vi "generate_DAC_voltages_flexRIO.vi"(7 "focus mode?":bool, 8 "derived values":T1, 9 "scan specification":T4={"x amplitude"=0, "x resolution (pixels)"=0, "x offset fly-forward (iterations)"=0, "x offset fly-back (iterations)"=0, "y resolution (nr. of lines)"=0, "y step size"=0, "iterations per pixel"=0, "number of frames"=0, "y offset (pixels)"=0, "number of y-brake lines  (before y-fly-back)"=0, "number y-brake lines (after y-fly-back)"=0, "number of y-fly-back steps"=8, "lines per z step"=0, "number of z/intensity tuples"=0, "number of repetitions (volumes or planes)"=0}, 10 "counter cluster in":T2, 11 "resonant trigger":bool) -> (0 "acquire?":bool, 1 "fly-back acquisition phase?":bool, 2 "counter cluster out":T2, 3 "DAC voltages":T3 {"ch6" max=4095 step=1; "ch5" max=4095 step=1; "ch4" max=4095 step=1; "ch3" max=4095 step=1; "ch2" max=4095 step=1; "ch1" max=4095 step=1; "ch0" max=4095 step=1})   [LabVIEW 2010]
uses:
  scan_specification_cluster_flexRIO.ctl
  DAC_voltage_cluster_flexRIO.ctl
  counter_cluster_flexRIO.ctl
  derived_values_cluster_flexRIO.ctl
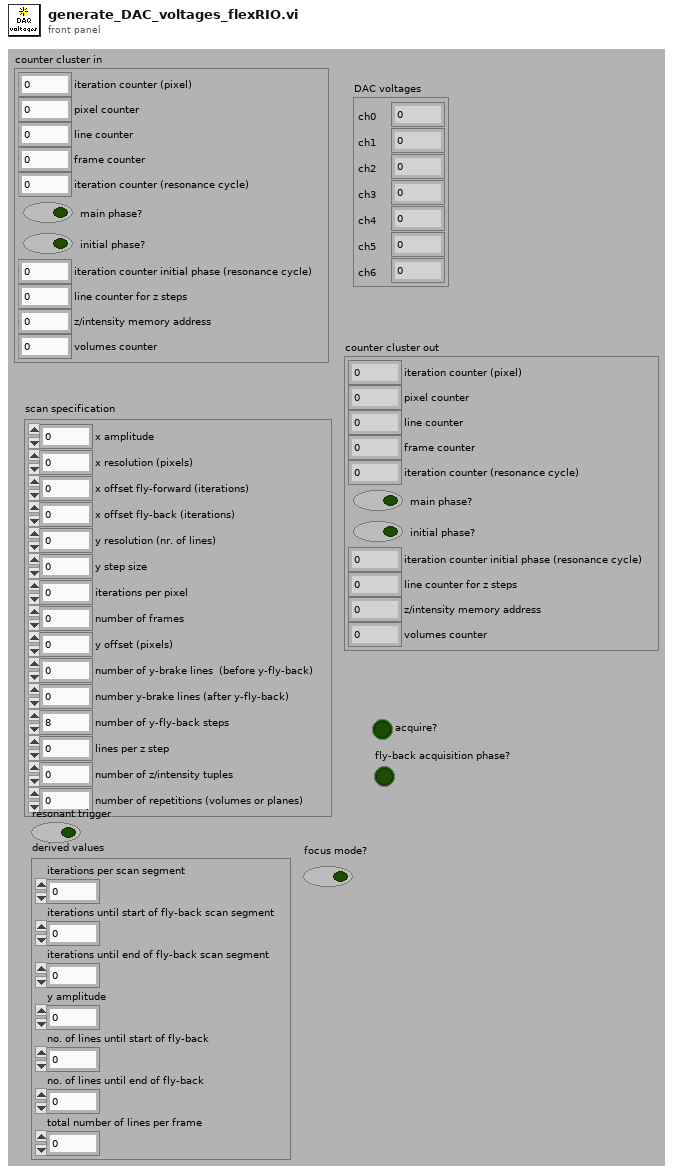
[diagram p1: front panel]
types:
  T1 = typedef "derived_values_cluster_flexRIO.ctl" = cluster{"iterations per scan segment":u16, "iterations until start of fly-back scan segment":u16, "iterations until end of fly-back scan segment":u16, "y amplitude":u16, "no. of lines until start of fly-back":u16, "no. of lines until end of fly-back":u16, "total number of lines per frame ":u16}
  T2 = typedef "counter_cluster_flexRIO.ctl" = cluster{"iteration counter (pixel)":u16, "pixel counter":u16, "line counter":u16, "frame counter":u16, "iteration counter (resonance cycle)":u16, "main phase?":bool, "initial phase?":bool, "iteration counter initial phase (resonance cycle)":u16, "line counter for z steps":u16, "z/intensity memory address":u32, "volumes counter":u16}
  T3 = typedef "DAC_voltage_cluster_flexRIO.ctl" = cluster{"ch0":u16, "ch1":u16, "ch2":u16, "ch3":u16, "ch4":u16, "ch5":u16, "ch6":u16}
  T4 = typedef "scan_specification_cluster_flexRIO.ctl" = cluster{"x amplitude":u16, "x resolution (pixels)":u16, "x offset fly-forward (iterations)":u16, "x offset fly-back (iterations)":u16, "y resolution (nr. of lines)":u16, "y step size":u16, "iterations per pixel":u16, "number of frames":i32, "y offset (pixels)":u16, "number of y-brake lines  (before y-fly-back)":u16, "number y-brake lines (after y-fly-back)":u16, "number of y-fly-back steps":u16, "lines per z step":u16, "number of z/intensity tuples":u16, "number of repetitions (volumes or planes)":i32}
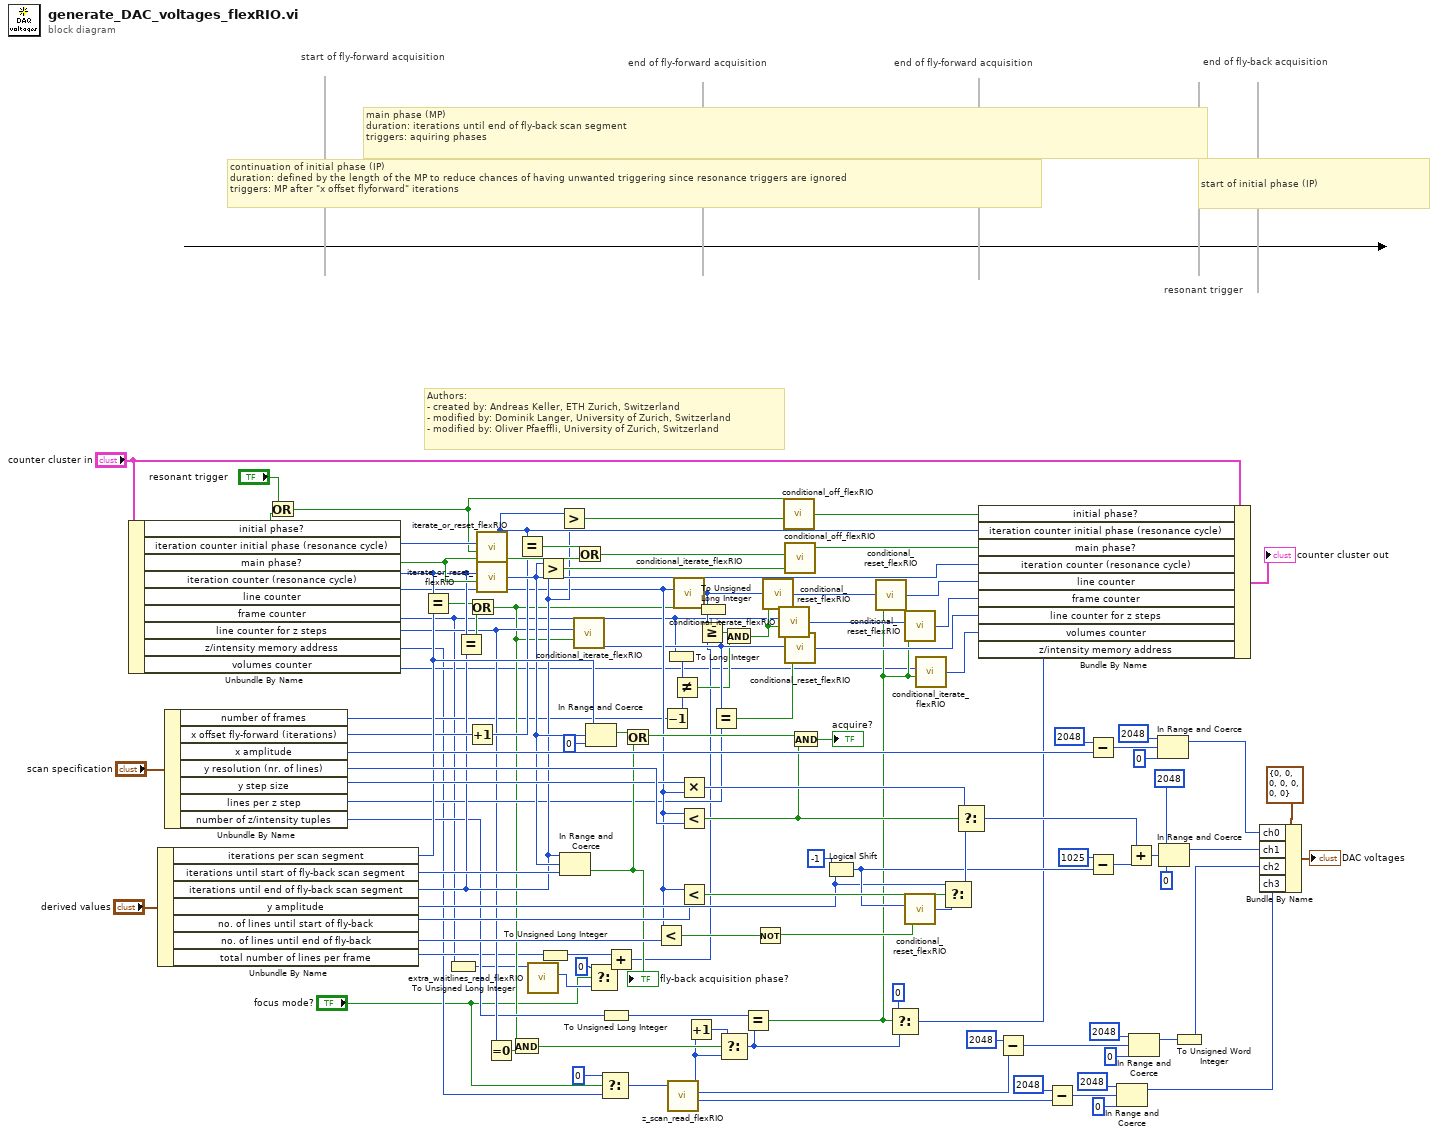
[diagram p0: block diagram]
diagram:
  # "start of initial phase (IP)"
  # "continuation of initial phase (IP)\nduration: defined by the length of the MP to reduce chances of having unwanted triggering since resonance triggers are ignored\ntriggers: MP after \"x offset flyforward\" iterations"
  # "end of fly-back acquisition"
  # "end of fly-forward acquisition"
  # "end of fly-forward acquisition"
  # "start of fly-forward acquisition"
  # "main phase (MP)\nduration: iterations until end of fly-back scan segment\ntriggers: aquiring phases"
  # "resonant trigger"
  # "Authors: \n- created by: Andreas Keller, ETH Zurich, Switzerland\n- modified by: Dominik Langer, University of Zurich, Switzerland\n- modified by: Oliver Pfaeffli, University of Zurich, Switzerland"
  n1 = Unbundle By Name("counter cluster in") -> ("initial phase?"=w85:bool, "iteration counter initial phase (resonance cycle)"=w81:u16, "main phase?"=w80:bool, "iteration counter (resonance cycle)"=w63:u16, "line counter"=w60:u16, "frame counter"=w14:u16, "line counter for z steps"=w53:u16, "z/intensity memory address"=w5:u32, "volumes counter"=w7:u16)
  n2 = Unbundle By Name("derived values") -> ("iterations per scan segment"=w83:u16, "iterations until start of fly-back scan segment"=w87:u16, "iterations until end of fly-back scan segment"=w62:u16, "y amplitude"=w69:u16, "no. of lines until start of fly-back"=w68:u16, "no. of lines until end of fly-back"=w86:u16, "total number of lines per frame"=w29:u16)
  n3 = Unbundle By Name("scan specification") -> ("number of frames"=w17:i32, "x offset fly-forward (iterations)"=w67:u16, "x amplitude"=w96:u16, "y resolution (nr. of lines)"=w93:u16, "y step size"=w92:u16, "lines per z step"=w57:u16, "number of z/intensity tuples"=w51:u16)
  n4 = Or(x="resonant trigger", y=w85) -> (x .or. y?=w77:bool)
  n5 = Equal?(x=w63, y=w83) -> (x = y?=w58:bool)
  n6 = To Unsigned Long Integer(number=w14) -> (unsigned 32bit integer=w30:u32)
  n7 = Equal?(x=w63, y=w62) -> (x = y?=w61:bool)
  n8 = Increment(x=w67) -> (x+1=w66:u16)
  n9 = Or(x=w58, y=w61) -> (x .or. y?=w35:bool)
  n10 = call "iterate_or_reset_flexRIO.vi"("iterate?"=w77, "number in"=w81) -> ("number out"=w64:u16)  [unwired: 4 in]
  n11 = call "iterate_or_reset_flexRIO.vi"("iterate?"=w80, "number in"=w63) -> ("number out"=w79:u16)  [unwired: 4 in]
  n12 = Equal To 0?(x=w53) -> (x = 0?=w36:bool)
  n13 = And(x=w35, y=w36) -> (x .and. y?=w34:bool)
  n14 = Equal?(x=w64, y=w66) -> (x = y?=w78:bool)
  n15 = call "extra_waitlines_read_flexRIO.vi"("address extra waitlines IN"=w30) -> ("extra waitline data"=w10:u32)  [unwired: 9 in, 1 out]
  n16 = Greater?(x=w79, y=w62) -> (0:w75:bool)
  n17 = To Unsigned Long Integer(number=w29) -> (unsigned 32bit integer=w28:u32)
  n18 = Greater?(x=w64, y=w62) -> (0:w65:bool)
  n19 = In Range and Coerce(upper limit=w62, x=w79, lower limit=w87) -> (In Range?=w59:bool)  [unwired: 1 out]
  "fly-back acquisition phase?" <- w59
  n20 = call "conditional_iterate_flexRIO.vi"("iterate?"=w35, "number in"=w53) -> ("number out"=w54:u16)  [unwired: 4 in]
  n21 = Or(x=w78, y=w80) -> (x .or. y?=w74:bool)
  n22 = In Range and Coerce(upper limit=w83, x=w79, lower limit=u16 0) -> (In Range?=w108:bool)  [unwired: 1 out]
  n23 = Select(t=u32 0, s="focus mode?", f=w10) -> (s? t:f=w9:u32)
  n24 = Select(t=u32 0, s="focus mode?", f=w5) -> (s? t:f=w4:u32)
  n25 = To Unsigned Long Integer(number=w51) -> (unsigned 32bit integer=w50:u32)
  n26 = Add(x=w28, y=w9) -> (x+y=w11:u32)
  n27 = Or(x=w108, y=w59) -> (x .or. y?=w91:bool)
  n28 = Less?(x=w60, y=w86) -> (x < y?=w89:bool)
  n29 = Decrement(x=w17) -> (x-1=w16:i32)
  n30 = To Long Integer(number=w14) -> (32bit integer=w13:i32)
  n31 = call "z_scan_read_flexRIO.vi"("address in"=w4) -> ("intensity"=w33:u16, "z-value"=w31:i16, "address out"=w32:u32)  [unwired: 8 in]
  n32 = Not Equal?(x=w13, y=w16) -> (x != y?=w15:bool)
  n33 = call "conditional_iterate_flexRIO.vi"("iterate?"=w35, "number in"=w60) -> ("number out"=w27:u16)  [unwired: 4 in]
  n34 = Multiply(x=w92, y=w60) -> (x*y=w112:u16)
  n35 = Less?(x=w60, y=w93) -> (x < y?=w90:bool)
  n36 = Less?(x=w60, y=w68) -> (x < y?=w114:bool)
  n37 = Increment(x=w32) -> (x+1=w52:u32)
  n38 = To Unsigned Long Integer(number=w27) -> (unsigned 32bit integer=w26:u32)
  n39 = Greater Or Equal?(x=w26, y=w11) -> (x >= y?=w19:bool)
  n40 = Equal?(x=w54, y=w57) -> (x = y?=w55:bool)
  n41 = Select(t=w52, s=w34, f=w32) -> (s? t:f=w49:u32)
  n42 = And(x=w19, y=w15) -> (x .and. y?=w18:bool)
  n43 = Equal?(x=w50, y=w49) -> (x = y?=w12:bool)
  n44 = Not(x=w89) -> (.not. x?=w71:bool)
  n45 = call "conditional_reset_flexRIO.vi"("reset?"=w18, "number in"=w27) -> ("number out"=w21:u16)  [unwired: 4 in]
  n46 = call "conditional_iterate_flexRIO.vi"("iterate?"=w18, "number in"=w14) -> ("number out"=w23:u16)  [unwired: 4 in]
  n47 = call "conditional_off_flexRIO.vi"("switch off?"=w65, "boolean in"=w77) -> ("boolean out"=w76:bool)  [unwired: 4 in]
  n48 = call "conditional_off_flexRIO.vi"("switch off?"=w75, "boolean in"=w74) -> ("boolean out"=w73:bool)  [unwired: 4 in]
  n49 = call "conditional_reset_flexRIO.vi"("reset?"=w55, "number in"=w54) -> ("number out"=w56:u16)  [unwired: 4 in]
  n50 = And(x=w91, y=w90) -> (x .and. y?=→"acquire?":bool)
  n51 = Logical Shift(y=i16 -1 ("n"), x=w69) -> (x << y=w72:u16)
  n52 = call "conditional_reset_flexRIO.vi"("reset?"=w12, "number in"=w21) -> ("number out"=w20:u16)  [unwired: 4 in]
  n53 = Select(t=u32 0, s=w12, f=w49) -> (s? t:f=w25:u32)
  n54 = call "conditional_reset_flexRIO.vi"("reset?"=w12, "number in"=w23) -> ("number out"=w24:u16)  [unwired: 4 in]
  n55 = call "conditional_reset_flexRIO.vi"("reset?"=w71, "number in"=w72) -> ("number out"=w70:u16)  [unwired: 4 in]
  n56 = call "conditional_iterate_flexRIO.vi"("iterate?"=w12, "number in"=w7) -> ("number out"=w22:u16)  [unwired: 4 in]
  n57 = Select(t=w69, s=w114, f=w70) -> (s? t:f=w113:u16)
  n58 = Select(t=w112, s=w90, f=w113) -> (s? t:f=w94:u16)
  n59 = Bundle By Name(cluster="counter cluster in", "initial phase?"=w76, "iteration counter initial phase (resonance cycle)"=w64, "main phase?"=w73, "iteration counter (resonance cycle)"=w79, "line counter"=w20, "frame counter"=w24, "line counter for z steps"=w56, "volumes counter"=w22, "z/intensity memory address"=w25) -> (→"counter cluster out":T2)
  n60 = Subtract(x=i16 2048, y=w31) -> (x-y=w41:i16)
  n61 = Subtract(x=u16 2048, y=w33) -> (x-y=w45:u16)
  n62 = Subtract(x=u16 2048, y=w96) -> (x-y=w100:u16)
  n63 = Subtract(x=u16 1025, y=w72) -> (x-y=w107:u16)
  n64 = In Range and Coerce(upper limit=u16 2048, x=w45, lower limit=u16 0) -> (coerced(x)=w43:u16)  [unwired: 1 out]
  n65 = Add(x=w94, y=w107) -> (x+y=w103:u16)
  n66 = In Range and Coerce(upper limit=i16 2048, x=w41, lower limit=i16 0) -> (coerced(x)=w38:i16)  [unwired: 1 out]
  n67 = In Range and Coerce(upper limit=u16 2048, x=w100, lower limit=u16 0) -> (coerced(x)=w99:u16)  [unwired: 1 out]
  n68 = In Range and Coerce(upper limit=u16 2048, x=w103, lower limit=u16 0) -> (coerced(x)=w102:u16)  [unwired: 1 out]
  n69 = To Unsigned Word Integer(number=w38) -> (unsigned 16bit integer=w37:u16)
  n70 = Bundle By Name(cluster=T3 {"ch0"=0, "ch1"=0, "ch2"=0, "ch3"=0, "ch4"=0, "ch5"=0, "ch6"=0} ("DAC voltages"), "ch0"=w99, "ch1"=w102, "ch2"=w37, "ch3"=w43) -> (→"DAC voltages":T3)
